vi "QuestionGui.vi"(8 "error in":errorcluster, 10 "Message":string) -> (0 "error out":errorcluster, 2 "ok?":bool)   [LabVIEW 2019, in "Tools.lvlib"]
uses:
  Tools.lvlib
  controls/buttons/OK.ctl
  controls/buttons/Cancel.ctl
  Message/MessageGui.Action.ctl
panel:
  in  "Cancel Button":T1
  out "_loop":i32(ring)=4
  in  "OKButton":T2
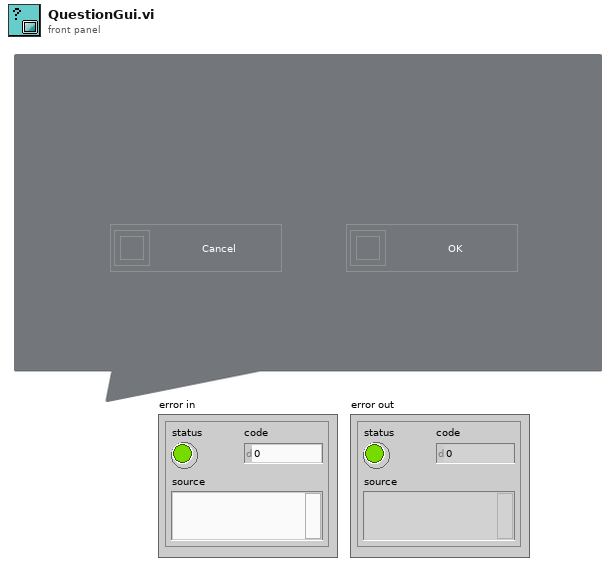
[diagram p1: front panel]
types:
  T1 = typedef "Tools.lvlib/Cancel.ctl" = bool
  T2 = typedef "Tools.lvlib/OK.ctl" = bool
  T3 = typedef "Tools.lvlib/MessageGui.Action.ctl" = enum32{"idle", "constructor", "destructor", "--- MessageGUI ---", "Gui.Translate"}
  T4 = enum32{"invalid app kind", "Development System", "Run Time System", "Student Edition", "Embedded LabVIEW", "Evaluation", "Custom"}
  T5 = typedef "LVPositionTypeDef.ctl" = cluster{"Left":i32, "Top":i32}
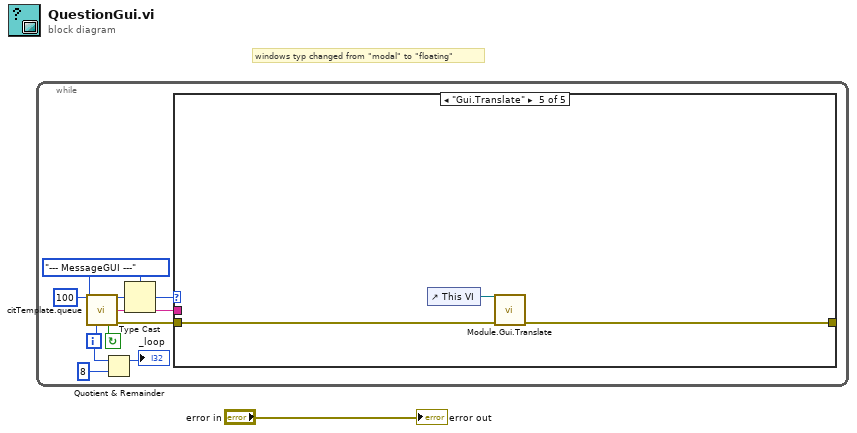
[diagram p0: block diagram]
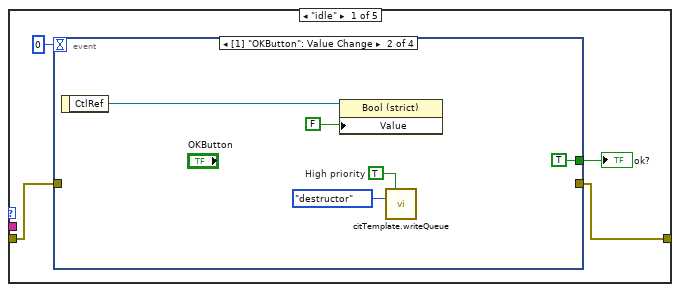
[diagram p2: hidden frame]
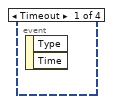
[diagram p3: hidden frame]
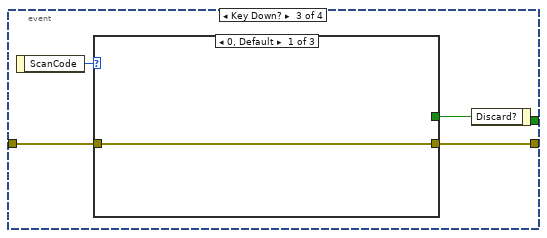
[diagram p4: hidden frame]
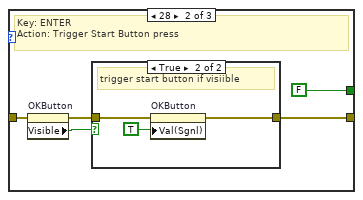
[diagram p5: hidden frame]
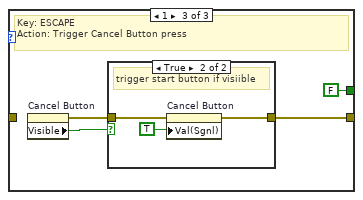
[diagram p7: hidden frame]
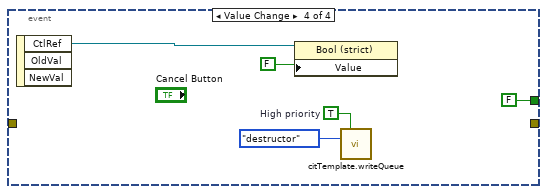
[diagram p9: hidden frame]
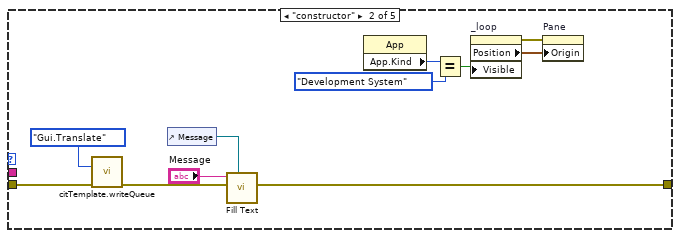
[diagram p10: hidden frame]
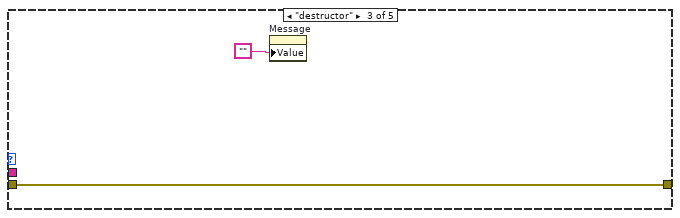
[diagram p11: hidden frame]
diagram:
  # "windows typ changed from \"modal\" to \"floating\""
  n1 = while {
    i -> [w2]
    stop <- w11 continue-if-true
    w5 = MessageGui.Action."--- MessageGUI ---" ("Action")
    n2 = call "citTemplate.queue.vi"("ms timeout (250 ms)"=100, "event enum"=w5, "iteration (-1)"=w2) -> ("event out"=w9:u32, "(flatten) data out"=w6:string, "continue"=w11:bool, "error out"=w7:errorcluster)  [unwired: 2 in, 7 out]
    n3 = Quotient & Remainder(x=w2, y=8) -> (x-y*floor(x/y)=→"_loop":i32)  [unwired: 1 out]
    n4 = Type Cast(type=w5, x=w9) -> (*(type *) &x=w8:T3)
    n5 = case shown="\"Gui.Translate\"" w8 {
      tunnel: w7 -> [w13 w52 w59 w61 w63]
      tunnel: w6 -> [_ _ _ _ _]
      tunnel: [w12 w50 w59 w61 w62] -> _
      frame "idle" {
        n6 = event shown="[1] \"OKButton\": Value Change" {
          selector: _ -> [_ _ _ _]
          dyn-events: _ -> [_ _ _ _]
          timeout: 0 -> [_ _ _ _]
          tunnel: [_ TRUE _ FALSE] -> w14
          tunnel: w13 -> [_ _ w22 _]
          tunnel: [_ _ w21 _] -> w12
          event Timeout {
            n7 = event-data() -> ()  [unwired: 3 out]
          }
          event Value Change {
            w16 = TRUE  # High priority
            n8 = event-data() -> ("CtlRef"=w19:refnum<vi>)  [unwired: 1 out]
            n9 = property class="Bool (strict)"(reference=w19, "Value"=T2 FALSE) -> ()  [unwired: 1 in, 2 out]
            n10 = call "citTemplate.writeQueue.vi"("High priority (F)"=w16, "event in (if not connected:all statemachine with data event)"=MessageGui.Action."destructor" ("Action")) -> ()  [unwired: 3 in, 11 out]
          }
          event Key Down? {
            n11 = event-data() -> ("ScanCode"=w24:i16)  [unwired: 1 out]
            n12 = case shown="0, Default" w24 {
              tunnel: [_ FALSE ("Discard?") FALSE ("Discard?")] -> w23
              tunnel: [w25 w29 w37] -> w21
              tunnel: w22 -> [w25 w26 _]
              frame 0, Default {
              }
              frame 28 {
                # "Key: ENTER\nAction: Trigger Start Button press"
                n13 = property on="OKButton" class="Bool (strict)"(error in=w26) -> (error out=w28:errorcluster, "Visible"=w27:bool)  [unwired: 1 in, 1 out]
                n14 = case shown="True" w27 {
                  tunnel: [w31 w34] -> w29
                  tunnel: w28 -> [w31 w33]
                  frame False {
                    # "Start button not visible, do nothing"
                  }
                  frame True {
                    # "trigger start button if visiible"
                    n15 = property on="OKButton" class="Bool (strict)"(error in=w33, "Val(Sgnl)"=TRUE) -> (error out=w34:errorcluster)  [unwired: 1 in, 1 out]
                  }
                }
              }
              frame 1 {
                # "Key: ESCAPE\nAction: Trigger Cancel Button press"
                n16 = property on="Cancel Button" class="Bool (strict)"() -> (error out=w36:errorcluster, "Visible"=w35:bool)  [unwired: 2 in, 1 out]
                n17 = case shown="True" w35 {
                  tunnel: [w39 w42] -> w37
                  tunnel: w36 -> [w39 w41]
                  frame False {
                    # "Start button not visible, do nothing"
                  }
                  frame True {
                    # "trigger start button if visiible"
                    n18 = property on="Cancel Button" class="Bool (strict)"(error in=w41, "Val(Sgnl)"=TRUE) -> (error out=w42:errorcluster)  [unwired: 1 in, 1 out]
                  }
                }
              }
            }
            n19 = event-data("Discard?"=w23) -> ()  [unwired: 1 in, 1 out]
          }
          event Value Change {
            w43 = TRUE  # High priority
            n20 = event-data() -> ("CtlRef"=w46:refnum<vi>)  [unwired: 3 out]
            n21 = property class="Bool (strict)"(reference=w46, "Value"=T2 FALSE) -> ()  [unwired: 1 in, 2 out]
            n22 = call "citTemplate.writeQueue.vi"("High priority (F)"=w43, "event in (if not connected:all statemachine with data event)"=MessageGui.Action."destructor" ("Action")) -> ()  [unwired: 3 in, 11 out]
          }
        }
        "ok?" <- w14
      }
      frame "constructor" {
        n23 = call "citTemplate.writeQueue.vi"("event in (if not connected:all statemachine with data event)"=MessageGui.Action."Gui.Translate" ("Action"), "error in (no error)"=w52) -> ("error out"=w51:errorcluster)  [unwired: 13 in]
        n24 = control-ref of="Message"() -> (w48:refnum<vi>)
        n25 = call "Fill Text.vi"("String ref"=w48, "Error In"=w51, "String in"="Message") -> ("Error Out"=w50:errorcluster)  [unwired: 8 in]
        n26 = property class="App"() -> ("App.Kind"=w56:T4)  [unwired: 2 in, 2 out]
        n27 = Equal?(x=w56, y=T4."Development System") -> (x = y?=w54:bool)
        n28 = property on="_loop" class="Ring (strict)"("Visible"=w54) -> (error out=w57:errorcluster, "Position"=w58:T5)  [unwired: 2 in, 1 out]
        n29 = property on="Pane" class="Pane"(error in=w57, "Origin"=w58) -> ()  [unwired: 1 in, 2 out]
      }
      frame "destructor" {
        n30 = property on="Message" class="Str"("Value"="") -> ()  [unwired: 2 in, 2 out]
      }
      frame "--- MessageGUI ---" {
      }
      frame "Gui.Translate" {
        n31 = control-ref of="This VI"() -> (w64:refnum<vi>)
        n32 = call "Module.Gui.Translate.vi"("error in"=w63, "VI ref in"=w64) -> ("error out"=w62:errorcluster)  [unwired: 7 in, 2 out]
      }
    }
  }
  "error out" <- "error in"
